vi "Binomial Noise Waveform.vi"(6 "sampling info":cluster{"Fs":dbl, "#s":dbl}={"Fs"=1000.0, "#s"=1000.0} {"Fs" format="%.2p"}, 7 "reset signal":bool, 8 "error in (no error)":errorcluster, 9 "trials":i32=1, 10 "seed":i32=-1, 11 "trial probability":dbl=0.5 format="%.2f") -> (0 "error out":errorcluster, 3 "signal out":waveform(u32))   [LabVIEW 2020, in "NI_MABase.lvlib"]
doc: "Generates a binomially-distributed pseudorandom pattern whose values are the number of occurrences of an event given the probability of that event occurring and the number of trials."
uses:
  NI_MABase.lvlib
  NI_AALBase.lvlib
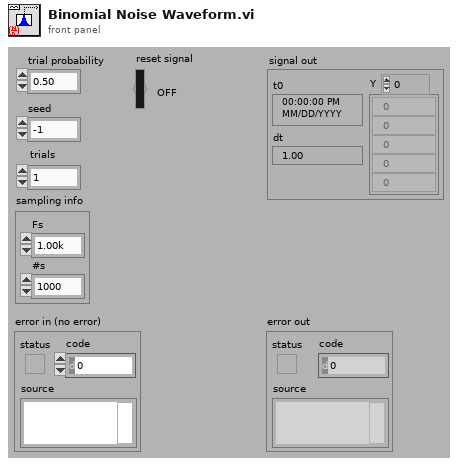
[diagram p1: front panel]
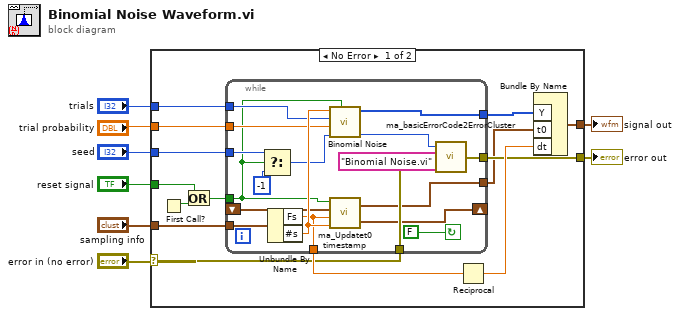
[diagram p0: block diagram]
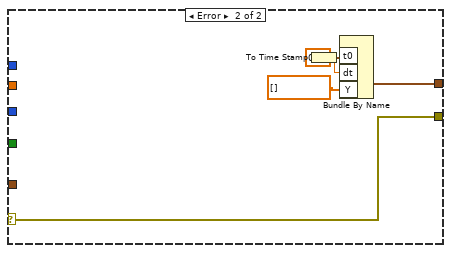
[diagram p2: hidden frame]
diagram:
  n1 = case shown="No Error" "error in (no error)" {
    selector: "error in (no error)" -> [w14 w45]
    tunnel: [w21 w45] -> w8
    tunnel: "sampling info" -> [w19 _]
    tunnel: "trial probability" -> [w17 _]
    tunnel: "seed" -> [w16 _]
    tunnel: [w15 w42] -> w3
    tunnel: "trials" -> [w13 _]
    tunnel: "reset signal" -> [w9 _]
    frame No Error {
      n2 = First Call?() -> (First Call?: T/F=w11:bool)
      n3 = Or(x=w9, y=w11) -> (x .or. y?=w10:bool)
      n4 = while {
        tunnel: w14 -> [w39]
        tunnel: w10 -> [w23]
        tunnel: w16 -> [w26]
        tunnel: w17 -> [w28]
        tunnel: [w31] -> w18
        tunnel: w19 -> [w32]
        tunnel: [w34] -> w20
        tunnel: [w35] -> w12
        shift-left: _ -> [w37]
        shift-right: [w36] -> _
        tunnel: [w38] -> w21
        tunnel: w13 -> [w27]
        stop <- FALSE continue-if-true
        n5 = Select(t=w26, s=w23, f=-1) -> (s? t:f=w24:i32)
        n6 = Unbundle By Name(w32) -> ("Fs"=w31:dbl, "#s"=w40:dbl)
        n7 = call "Binomial Noise.vi"("initialize?"=w23, "seed"=w24, "trial probability"=w28, "trials"=w27, "samples"=w40) -> ("error"=w30:i32, "binomial noise"=w34:u32[])  [unwired: 5 in]
        n8 = call "ma_Updatet0 timestamp.vi"("samples"=w40, "sampling rate (S/s)"=w31, "tf previous"=w37, "Reset Generation"=w23) -> ("tf new"=w36:timestamp, "t0"=w35:timestamp)
        n9 = call "ma_basicErrorCode2ErrorCluster.vi"("error in (no error)"=w39, "subVI name"="Binomial Noise.vi" ("subVI Name"), "Error Code"=w30) -> ("error out"=w38:errorcluster)
      }
      n10 = Reciprocal(x=w18) -> (1/x=w22:dbl)
      n11 = Bundle By Name("Y"=w20, "t0"=w12, "dt"=w22) -> (w15:waveform(u32))  [unwired: 1 out]
    }
    frame Error {
      w44 = 0.0 ("t0")
      n12 = To Time Stamp(1:w44) -> (0:w41:timestamp)
      n13 = Bundle By Name("t0"=w41, "dt"=w44, "Y"=dbl[] []) -> (w42:waveform(dbl))  [unwired: 1 out]
    }
  }
  "error out" <- w8
  "signal out" <- w3
